vi "NewtonsPSM_Conf_RMSMeter.vi"(0 "VISA session":refnum<visa-resource-name>, 9 "Low Blanking (Off)":bool, 11 "error in (no error)":errorcluster) -> (4 "dup VISA session":refnum<visa-resource-name>, 15 "error out":errorcluster)   [LabVIEW 2025, in "NewtonsPSM1735.lvlib"]
doc: "This VI set the RMS Voltmeter parameters to the PPA2530."
uses:
  NewtonsPSM1735.lvlib
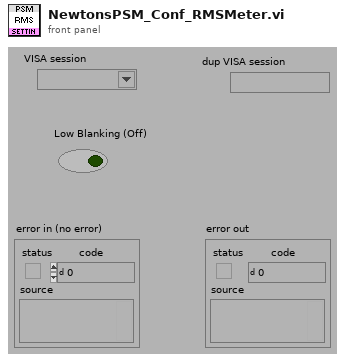
[diagram p1: front panel]
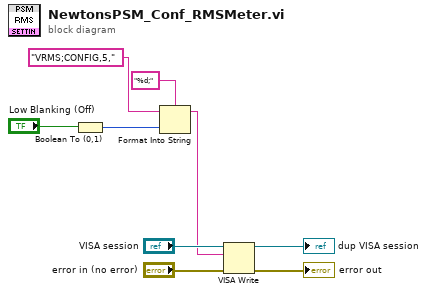
[diagram p0: block diagram]
diagram:
  n1 = Boolean To (0,1)(Boolean="Low Blanking (Off)") -> (0, 1=w1:i16)
  n2 = Format Into String(format string="%d;", initial string="VRMS;CONFIG,5,", w1) -> (resulting string=w3:string)  [unwired: 1 in, 1 out]
  n3 = VISA Write(VISA resource name="VISA session", write buffer=w3, error in (no error)="error in (no error)") -> (VISA resource name out=→"dup VISA session":refnum<visa-resource-name>, error out=→"error out":errorcluster)  [unwired: 1 out]
